vi "Global variables.vi"() -> ()   [LabVIEW 2012]
panel:
  in  "Measured Pos data":string
  in  "Target positions":string
  in  "Measurement Image":string
  in  "Monitoring image":string
  in  "Image Type (measurement)":T1 items=["Grayscale (U8)", "Grayscale (I16)", "Grayscale (SGL)", "Complex (CSG)", "RGB (U32)", "HSL (U32)", "RGB (U64)", "Grayscale (U16)"]
  in  "Image Type (monitoring)":T1 items=["Grayscale (U8)", "Grayscale (I16)", "Grayscale (SGL)", "Complex (CSG)", "RGB (U32)", "HSL (U32)", "RGB (U64)", "Grayscale (U16)"]
  in  "Measurement ROI":T2 {"Contours"."Type" items=["No Selection", "Point", "Line", "Rectangle", "Oval", "Polygon", "Freehand Region", "Annulus", "Unused2", "Unused3", "Broken Line", "Freehand Line", "Rotated Rectangle"]}
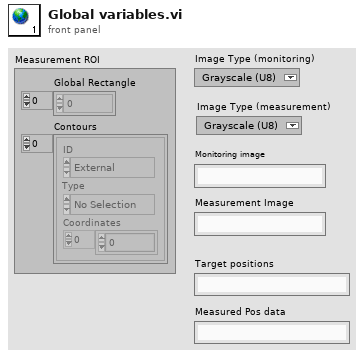
[diagram p1: front panel]
types:
  T1 = typedef "Image Type" = u32
  T2 = typedef "ROI Descriptor" = cluster{"Global Rectangle":i32[], "Contours":cluster{"ID":enum32{"External", "Internal"}, "Type":u32, "Coordinates":i32[]}[]}
diagram:
